vi "new_from_int.vi"(5 "Response in":refnum<class "Response.lvclass">, 8 "error in (no error)":errorcluster, 11 "response_ref":u64) -> (0 "error out":errorcluster, 3 "Response out":refnum<class "Response.lvclass">)   [LabVIEW 2020, in "Response.lvclass"]
uses:
  Response.lvclass
  Response.lvclass/Response.ctl
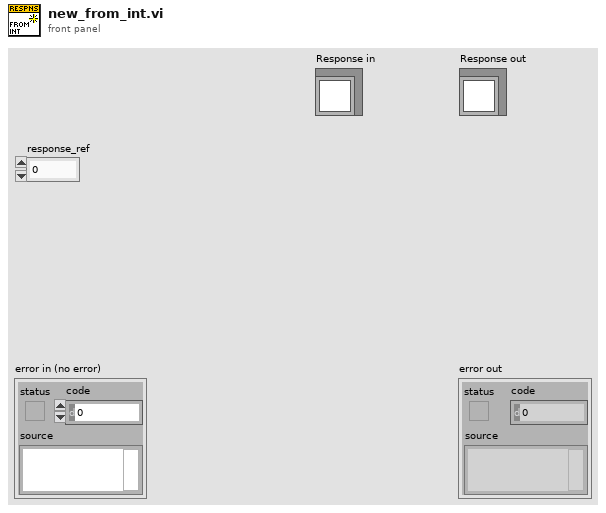
[diagram p1: front panel]
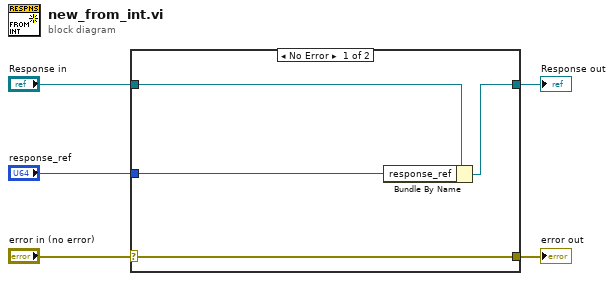
[diagram p0: block diagram]
diagram:
  n1 = case shown="No Error" "error in (no error)" {
    selector: "error in (no error)" -> [w9 w10]
    tunnel: [w9 w10] -> w4
    tunnel: [w7 w11] -> w2
    tunnel: "Response in" -> [w8 w11]
    tunnel: "response_ref" -> [w6 _]
    frame No Error {
      n2 = Bundle By Name(cluster=w8, "response_ref"=w6) -> (w7:refnum<class "Response.lvclass">)
    }
    frame Error {
    }
  }
  "error out" <- w4
  "Response out" <- w2
